vi "[Global]CamNumber.vi"() -> ()   [LabVIEW 2015]
panel:
  in  "Cam Number":i32=16
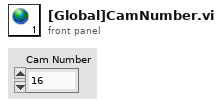
[diagram p1: front panel]
diagram:
